vi "Examen01.vi"() -> ()   [LabVIEW 2020]
uses:
  <vilib>/numeric/Random Number (Range) DBL.vi
panel:
  out "Waveform Chart":dynamicdata(graph)
  out "RANGO":bool
  out "N° LÍMITE MÁXIMO":dbl
  out "ON/OFF":bool
  out "SEÑAL ANALÓGICA SIN FILTRAR":dbl
  in  "PARO DEL CILCLO":bool
  # "DIEGO JÁUREGUI ONTIVEROS 3MM4"
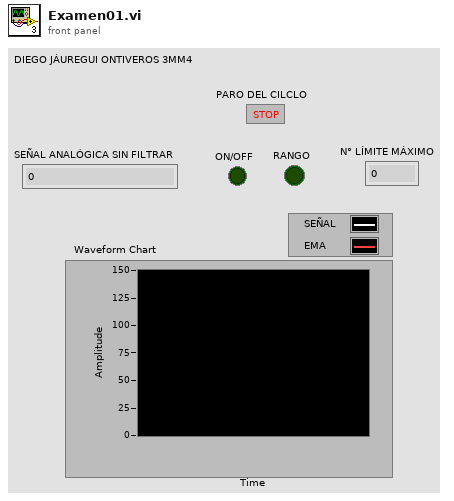
[diagram p1: front panel]
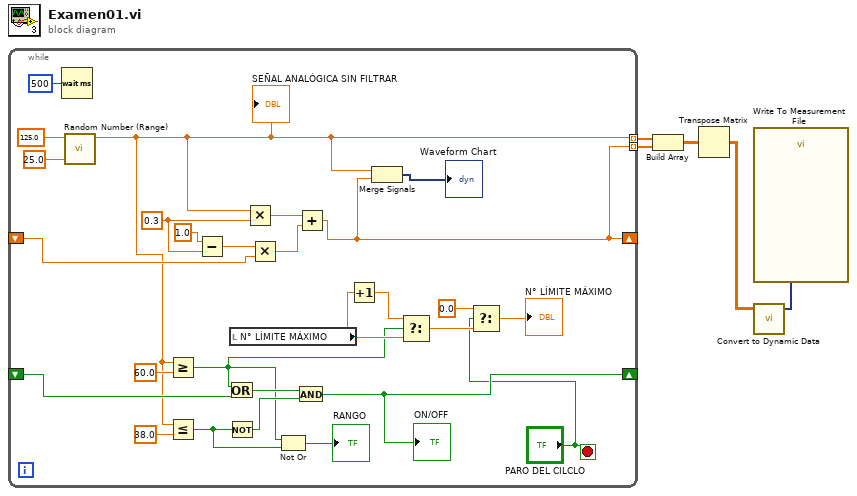
[diagram p0: block diagram]
diagram:
  n1 = while {
    shift-right: [w6] -> _
    shift-left: _ -> [w16]
    shift-right: [w14] -> _
    shift-left: _ -> [w15]
    tunnel: [w7] -> w5 mode=indexing
    tunnel: [w6] -> w4 mode=indexing
    stop <- "PARO DEL CILCLO" stop-if-true
    w29 = 0.3
    n2 = Wait (ms)(milliseconds to wait=u32 500) -> ()  [unwired: 1 out]
    n3 = call-poly <vilib>:"Random Number (Range).vi"("lower bound (0)"=25.0, "upper bound (100)"=125.0) -> ("number"=w7:dbl)  [unwired: 9 in]
    "SEÑAL ANALÓGICA SIN FILTRAR" <- w7
    n4 = Greater Or Equal?(x=w7, y=60.0) -> (x >= y?=w18:bool)
    n5 = Less Or Equal?(x=w7, y=38.0) -> (x <= y?=w17:bool)
    n6 = Subtract(x=1.0, y=w29) -> (x-y=w27:dbl)
    n7 = Or(x=w18, y=w15) -> (x .or. y?=w24:bool)
    n8 = Not(x=w17) -> (.not. x?=w25:bool)
    n9 = local read "N° LÍMITE MÁXIMO"() -> (w20:dbl)
    n10 = Multiply(x=w7, y=w29) -> (x*y=w26:dbl)
    n11 = Multiply(x=w27, y=w16) -> (x*y=w28:dbl)
    n12 = Not Or(1:w17, 2:w18) -> (0:→"RANGO":bool)
    n13 = And(x=w24, y=w25) -> (x .and. y?=w14:bool)
    "ON/OFF" <- w14
    n14 = Add(x=w26, y=w28) -> (x+y=w6:dbl)
    n15 = Increment(x=w20) -> (x+1=w21:dbl)
    n16 = Merge Signals(w7, w6) -> (→"Waveform Chart":dynamicdata)
    n17 = Select(t=w21, s=w18, f=w20) -> (s? t:f=w11:dbl)
    n18 = Select(t=0.0, s="PARO DEL CILCLO", f=w11) -> (s? t:f=→"N° LÍMITE MÁXIMO":dbl)
  }
  n19 = Build Array(w5, w4) -> (w1:dbl[][])
  n20 = Transpose Matrix(1:w1) -> (0:w3:dbl[][])
  n21 = call "Convert to Dynamic Data"("2D Array"=w3) -> ("Dynamic Data Type"=w2:dynamicdata)  [unwired: 3 in]
  n22 = call "Write To Measurement File"("Signals"=w2) -> ()  [unwired: 16 in, 3 out]
